vi "Calibrate_Thermocouples.vi"(4 "Save Data in":bool, 5 "Thermocouples":dbl[](array[numeric]), 6 "Tester in":string(combo)="J Singleton", 7 "reference":refnum<vi>, 9 "Override Build\nFile Write in":bool, 10 "reference 2":refnum<vi>, 11 "Queue in":refnum<queue>) -> (1 "Number in Queue 2":i32, 2 "Raw Data Directory Path 2":path, 3 "Raw Data File Path 2":path)   [LabVIEW 2017]
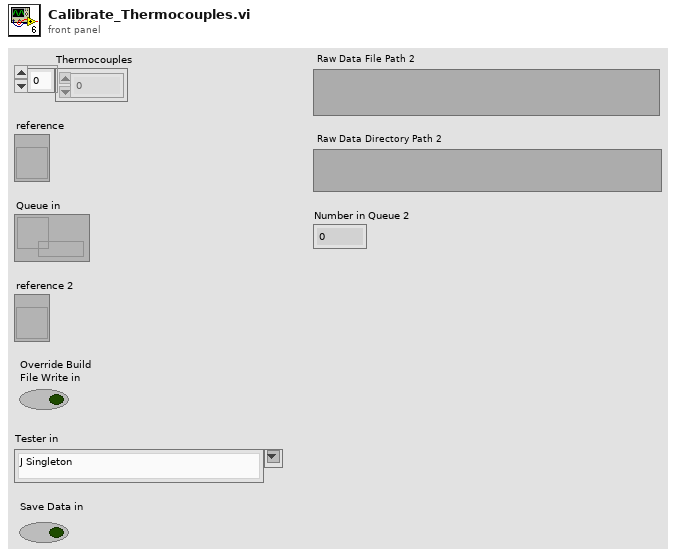
[diagram p1: front panel]
types:
  T1 = cluster{"Build Sheet Directory 2":path, "File Path":path, "Directory Path":path, "Build Number 2":string, "Tester in":string, "Purpose of Test (NO COMMAS) 2":string, "Test Comments (NO COMMAS)  2":string, "Test Request\n    Number 2":string, "Data Root Directory 2":path}
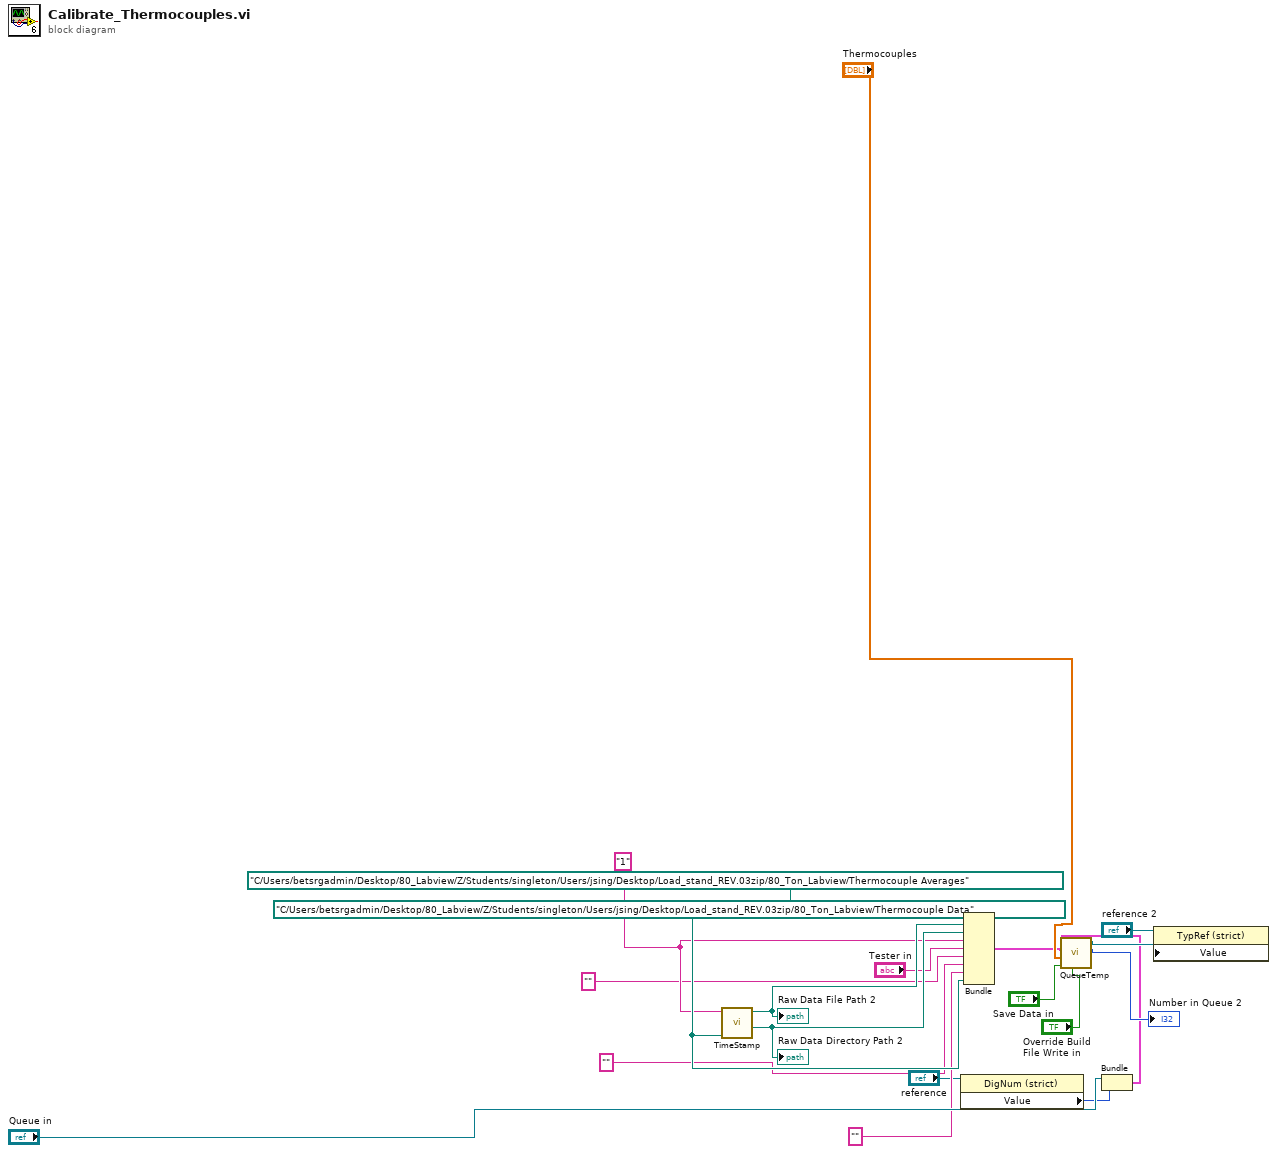
[diagram p0: block diagram]
diagram:
  w7 = "1" ("Build Number 2")
  w10 = path "C:/Users/betsrgadmin/Desktop/80_Labview/Z/Students/singleton/Users/jsing/Desktop/Load_stand_REV.03zip/80_Ton_Labview/Thermocouple Data" ("Data Root Directory 2")
  n1 = call "TimeStamp.vi"("Root Path"=w10, "Build Name"=w7) -> ("Directory Path"=w9:path, "File Path"=w8:path)  [unwired: 7 in, 1 out]
  "Raw Data Directory Path 2" <- w9
  "Raw Data File Path 2" <- w8
  n2 = property class="DigNum (strict)"(reference="reference") -> ("Value"=w12:i32)  [unwired: 1 in, 2 out]
  n3 = Bundle("Build Sheet Directory 2"=path "C:/Users/betsrgadmin/Desktop/80_Labview/Z/Students/singleton/Users/jsing/Desktop/Load_stand_REV.03zip/80_Ton_Labview/Thermocouple Averages", "File Path"=w8, "Directory Path"=w9, "Build Number 2"=w7, "Tester in"="Tester in", "Purpose of Test (NO COMMAS) 2"="", "Test Comments (NO COMMAS)  2"="", "Test Request\n    Number 2"="" ("Test Request\n    Number 2"), "Data Root Directory 2"=w10) -> (w14:T1)  [unwired: 1 in]
  n4 = Bundle("Queue in"="Queue in", "Value"=w12) -> (w13:cluster{"Queue in":refnum<queue>, "Value":i32})  [unwired: 1 in]
  n5 = call "QueueTemp.vi"("Override Build\nFile Write"="Override Build\nFile Write in", "Save Data"="Save Data in", "Data In"="Thermocouples", "Saving Cluster"=w14, "Cluster"=w13) -> ("Number in Queue"=→"Number in Queue 2":i32, "queue out"=w19:refnum<queue>)  [unwired: 5 in]
  n6 = property class="TypRef (strict)"(reference="reference 2", "Value"=w19) -> ()  [unwired: 1 in, 2 out]
